vi "Read End-of-File.vi"(8 "Error In":errorcluster, 11 "Channel In":refnum<class "Channel.lvclass">) -> (0 "Error Out":errorcluster, 2 "End-of-File?":bool, 3 "Channel Out":refnum<class "Channel.lvclass">)   [LabVIEW 2021, in "Field_RnD_Services_LIBSSH2_Toolkit.lvlib" / "Channel.lvclass"]
doc: "Determines if the remote SSH server is at the End-of-File (EOF)."
uses:
  Channel.lvclass
  Session/Session.lvclass
  Field_RnD_Services_LIBSSH2_Toolkit.lvlib
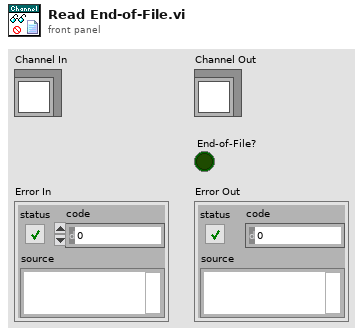
[diagram p1: front panel]
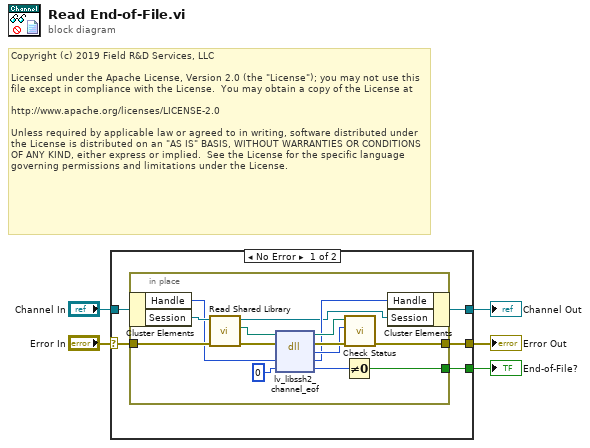
[diagram p0: block diagram]
diagram:
  # "Copyright (c) 2019 Field R&D Services, LLC\n\nLicensed under the Apache License, Version 2.0 (the \"License\"); you may not use this file except in compliance with the License.  You may obtain a copy of the License at\n\nhttp://www.apache.org/licenses/LICENSE-2.0\n\nUnless required by applicable law or agreed to in writing, software distributed under the License is distributed on an \"AS IS\" BASIS, WITHOUT WARRANTIES OR CONDITIONS OF ANY KIND, either express or implied.  See the License for the specific language governing permissions and limitations under the License."
  n1 = case shown="No Error" "Error In" {
    selector: "Error In" -> [w8 w26]
    tunnel: [w7 w26] -> w4
    tunnel: "Channel In" -> [w10 w25]
    tunnel: [w9 w25] -> w2
    tunnel: [w6 _] -> w1
    frame No Error {
      n2 = in-place {
        in-place-border: w8 -> [w21]
        in-place-border: [w17] -> w7
        in-place-border: [w11] -> w6
        n3 = in-place-cluster #1(w10) -> ("Handle"=w16:u64, "Session"=w24:refnum<class "Session.lvclass">)
        n4 = call "Read Shared Library.vi"("Error In"=w21, "Session In"=w24) -> ("Erorr Out"=w22:errorcluster, "libssh2lv Shared Library"=w23:path, "Session Out"=w14:refnum<class "Session.lvclass">)  [unwired: 7 in]
        n5 = dll-call lib="libssh2lv.*" fn="lv_libssh2_channel_eof"(path in=w23, error in=w22, "handle"=w16, "eof"=0) -> (path out=w19:path, error out=w20:errorcluster, "status"=w18:i32, "handle"=w15:u64, "eof"=w12:i32)  [unwired: 1 in]
        n6 = Not Equal To 0?(x=w12) -> (x != 0?=w11:bool)
        n7 = call "Check Status.vi"("Error In"=w20, "Status"=w18, "libssh2lv Shared Library In"=w19) -> ("Error Out"=w17:errorcluster)  [unwired: 7 in, 1 out]
        n8 = in-place-cluster #1("Handle"=w15, "Session"=w14) -> (w9:refnum<class "Channel.lvclass">)
      }
    }
    frame Error {
    }
  }
  "Error Out" <- w4
  "Channel Out" <- w2
  "End-of-File?" <- w1
